vi "PixelFly.vi"() -> ()   [LabVIEW 2012]
uses:
  <vilib>/Platform/TimedLoop/XDataNode/timing_clust.ctl
  <vilib>/Platform/TimedLoop/XDataNode/nitl_modes.ctl
  <vilib>/Platform/TimedLoop/XDataNode/wakeup.ctl
  <vilib>/platform/TimedLoop/XDataNode/XDataNode.xnode
  <vilib>/Platform/TimedLoop/XDataNode/XDNodeRunTimeDep.lvlib
panel:
  in  "Tab Control":enum32{"Control", "Advanced"}(tab)
  out "Intensity Graph":u16[][](graph)
  in  "?":u16(ring) items=["Debug", "Bulb Trigger", "Free Run"]
  in  "bUseBuffer0":bool
  in  "Open StructureIn":T1={"Size"=88, "InterfaceType"=0, "Camera Number"=0, "CameraNumAtInterface"=0, "OpenFlags"=[], "OpenDWFlags"=[], "OpenPtrs"=[]}
  in  "bUseBuffer1":bool
  in  "stop":bool
  in  "stop 2":bool
  out "BufNr0":i16
  out "BufNr1":i16
  out "Bits/pixel":u16
  in  "ROIX1":u16=1 min=1
  in  "ROIY1":u16=1 min=1
  in  "ROIY0":u16=1 min=1
  in  "ROIX0":u16=1 min=1
  in  "DelayTimeBase":u16(ring)=2 items=["nanoseconds", "microseconds", "milliseconds"]
  in  "ExposureTimeBase":u16(ring)=1 items=["nanoseconds", "microseconds", "milliseconds"]
  in  "Exposure":u32=60
  in  "InterfaceType":u16(ring)=6 items=["IEEE1394 - Firewire", "IEEE1394/Firewire", "Matrox Helios Camera Link", "Silicon Software ME3 Camera Link", "National Instruments Camera Link", "Gigabit Ethernet", "USB", "Reserved", "Reserved", "Reserved", "Generic Camera Link with CLSER.DLL"]
  in  "Rate":i32
  in  "StorageMode":bool
  in  "TriggerMode":u16(ring)=2 items=["Auto", "Software", "External sequence start ", "External exposure control"]
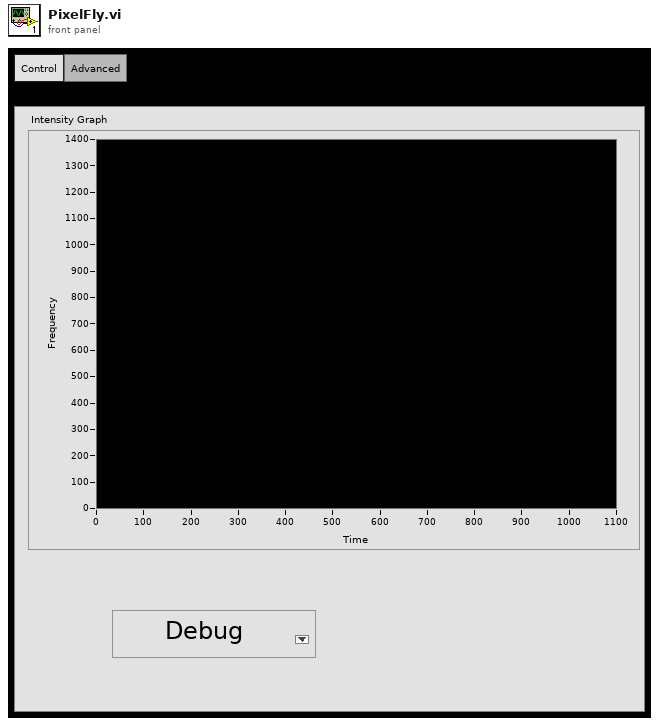
[diagram p1: front panel]
types:
  T1 = cluster{"Size":u16, "InterfaceType":u16, "Camera Number":u16, "CameraNumAtInterface":u16, "OpenFlags":u16[], "OpenDWFlags":u32[], "OpenPtrs":u32[]}
  T2 = typedef "XDNodeRunTimeDep.lvlib/timing_clust.ctl" = cluster{"Expected End [f-1]":u64, "Actual End [f-1]":u64, "Finished Late? [f-1]":bool, "Expected End [i-1]":u64, "Actual End [i-1]":u64, "Finished Late? [i-1]":bool, "Expected Start [i]":u64, "Actual Start [i]":u64, "Expected Start [f]":u64, "Actual Start [f]":u64, "Source Name":string, "Structure Name":string, "Period":i64, "Deadline":i64, "Offset":i64, "Start":i64, "Priority":i32, "Timeout":i32, "Mode":T3, "Wakeup Reason":T4, "Error":errorcluster, "Source Type":string, "Secondary Source Type":string, "Global End Time":u64, "Global Start Time":u64, "Frame Duration":u64, "Iteration Duration":u64, "Assigned CPU":i32, "I/O Scan Engine Mode":u32}
  T3 = typedef "XDNodeRunTimeDep.lvlib/nitl_modes.ctl" = enum32{"No Change", "Process missed periods, maintain original phase", "Discard missed periods, maintain original phase", "Process missed periods, ignore original phase", "Discard missed periods, ignore original phase"}
  T4 = typedef "XDNodeRunTimeDep.lvlib/wakeup.ctl" = enum32{"Normal", "Aborted", "Asynchronous wakeup", "Timing source error", "Timed loop error", "Timeout"}
  T5 = cluster{"Size":u16, "CamType":u16, "CamSubType":u16, "SerialNumber":u32, "HWVersion":u32, "FWVersion":u32, "InterfaceType":u16, "HardwareVersion":cluster{"BoardNum":u16, "HWVersions":cluster{"BoardName":string, "BatchNumber":u16, "MinorRevision":u8, "MajorRevision":u8, "Variant":u16}[]}, "FirmwareVersion":cluster{"DeviceNum":u16, "FWVersions":cluster{"DeviceName":string, "MinorRevision":u8, "MajorRevision":u8, "Variant":u16}[]}}
  T6 = cluster{"Size":u16, "SensorTypeDESC":u16, "SensorSubtypeDESC":u16, "MaxHorizontalResStdDESC":u16, "MaxVerticalResStdDESC":u16, "MaxHorizontalResExtDESC":u16, "MaxVerticalResExtDESC":u16, "DynResDESC":u16, "MaxBinHorzDESC":u16, "BinHorzStepDESC":bool, "MaxBinVertDESC":u16, "BinVertStepDESC":bool, "ROIHorzStepDESC":u16, "ROIVertStepDESC":u16, "NumADCDESC":u16, "IRDESC":bool, "MinDelayDESC":u32, "MaxDelayDESC":u32, "MinDelayStepDESC":u32, "MinExpoDESC":u32, "MaxExpoDESC":u32, "MinExpoStepDESC":u32, "MinDelayIRDESC":u32, "MaxDelayIRDESC":u32, "MinExpoIRDESC":u32, "MaxExpoIRDESC":u32, "TimeTableDESC":bool, "DoubleImageDESC":bool, "MinCoolSetDESC":i16, "MaxCoolSetDESC":i16, "MDefaultCoolSetDESC":i16, "PowerDownModeDESC":bool, "OffsetRegDESC":bool, "ColorPattern":cluster{"UpperLeftColor":u8, "UpperRightColor":u8, "LowerLeftColor":u8, "LowerRightColor":u8}, "PatternTypeDESC":bool, "PixelRates":u32[], "CoversionFactors":u16[], "Reserved":u32[], "NoiseFilterCapable":bool, "HotPixelCapable":bool, "HotPixelWithNoiseFilter":bool, "ASCIITimeCapable":bool, "Extended Description":bool, "Get Extended":bool, "Reserved Flag 1":bool, "Reserved Flag 2":bool}
  T7 = cluster{u16[][], "XResAct":u16, "YResAct":u16, "BufNrOut":i16, "BufNrOut":i16, "ErrorOut":errorcluster, "hout":u64, "Bits/pixel":u16}
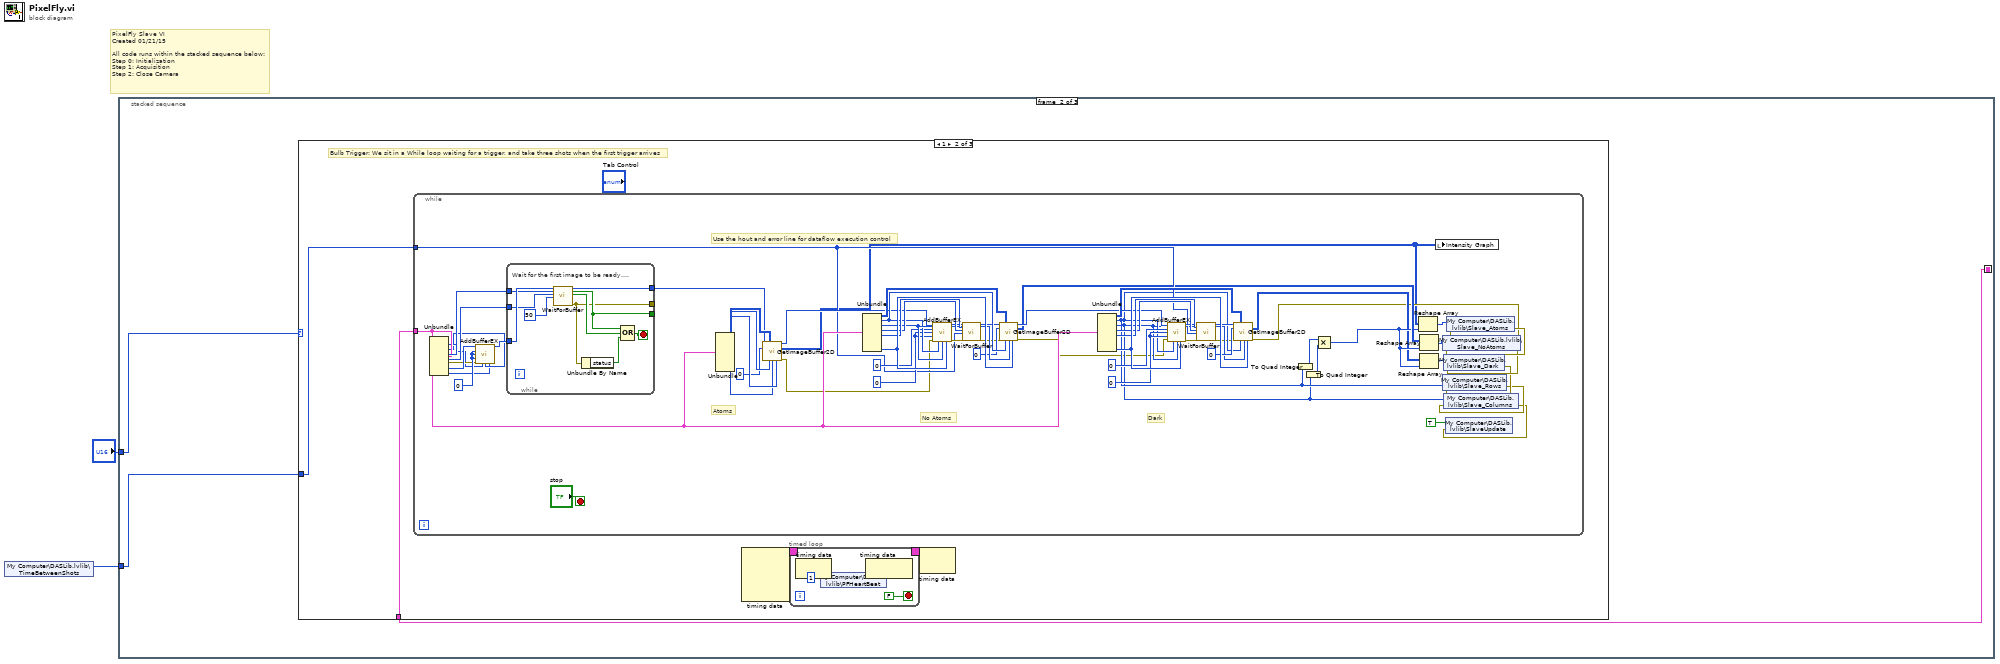
[diagram p0: block diagram]
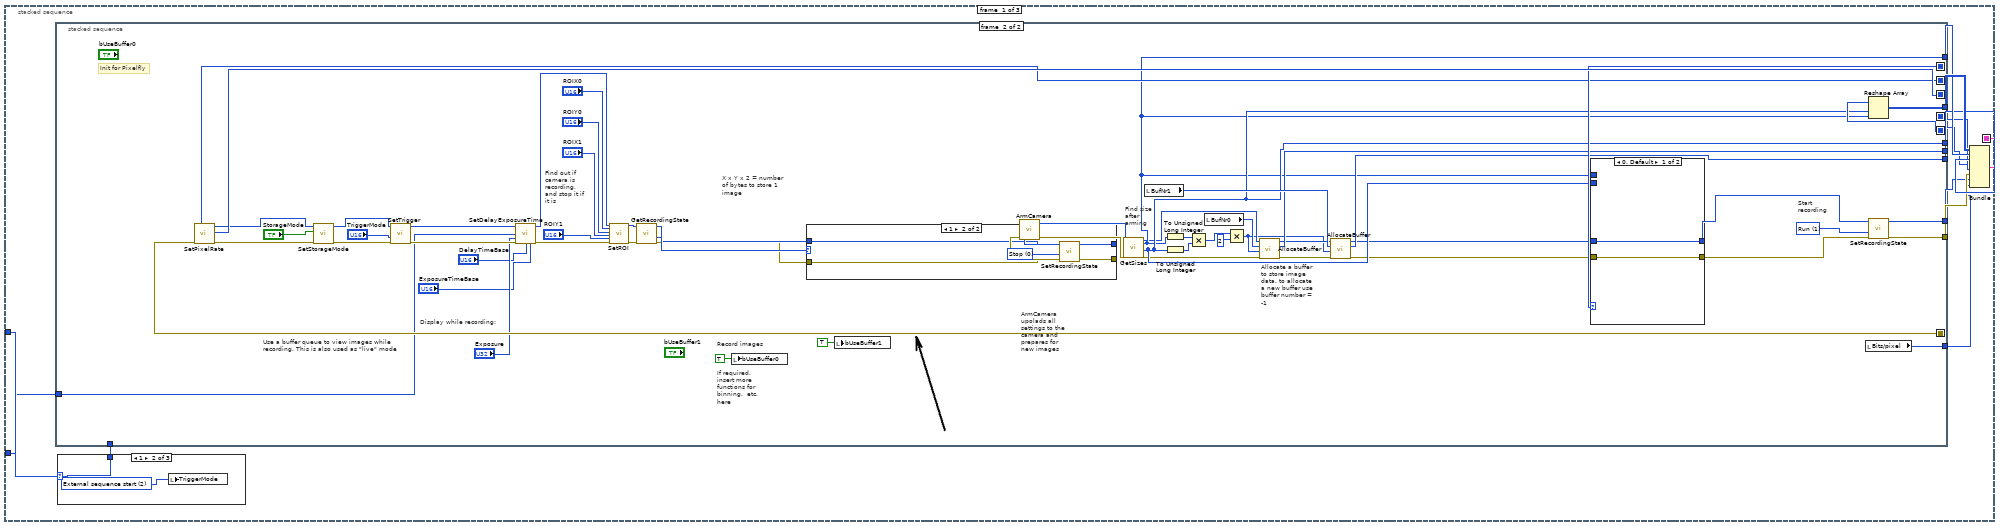
[diagram p2: hidden frame]
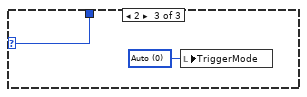
[diagram p4: hidden frame]
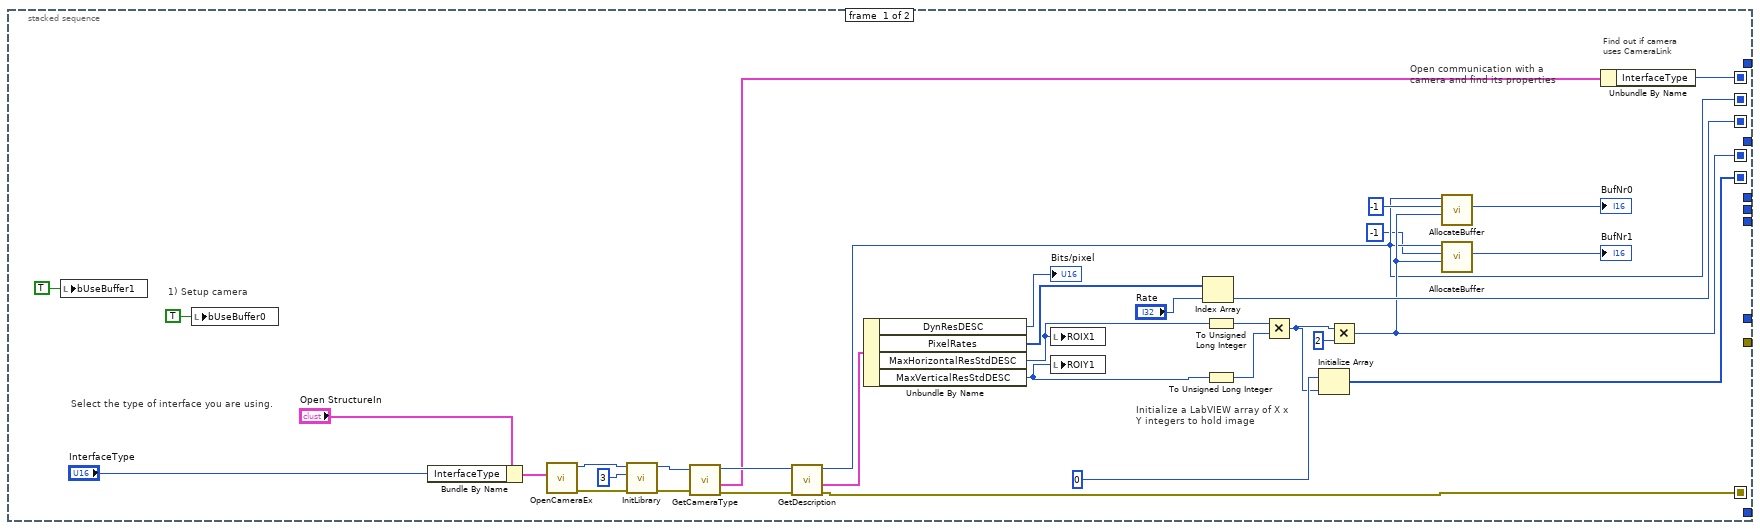
[diagram p5: hidden frame]
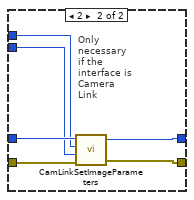
[diagram p6: hidden frame]
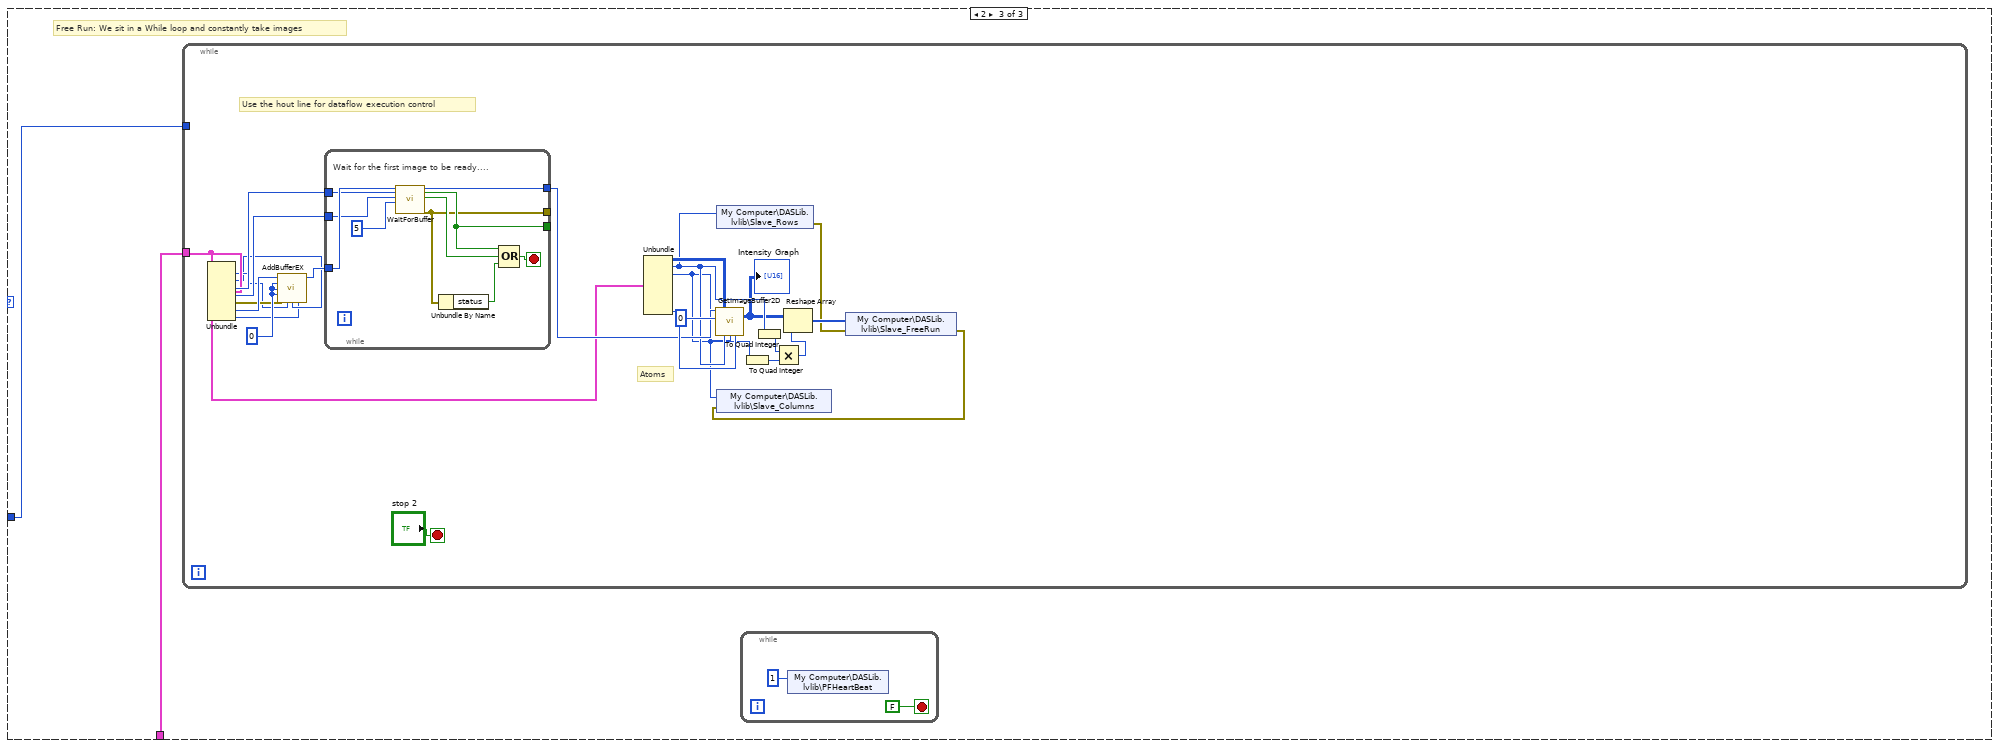
[diagram p9: hidden frame]
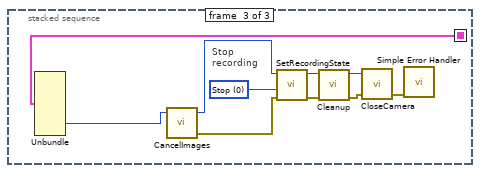
[diagram p10: hidden frame]
diagram:
  # "PixelFly Slave VI\nCreated 01/21/15\n\nAll code runs within the stacked sequence below:\nStep 0: Initialization\nStep 1: Acquisition\nStep 2: Close Camera"
  n1 = shared-variable "My Computer\\DASLib.lvlib\\TimeBetweenShots"() -> (w1:i64)  [unwired: 1 in, 1 out]
  n2 = stacked-sequence {
    seq-local: [w6 _ _] -> [_ w128 w253]
    tunnel: "?" -> [w5 w129 _]
    tunnel: w1 -> [w3 w127 _]
    frame #0 {
      n3 = case shown="1" w5 {
        selector: w5 -> [w15 w16 w18]
        tunnel: [w15 w16 w18] -> w4
        frame 0, Default {
        }
        frame 1 {
          w17 = u16 2 items=["Auto", "Software", "External sequence start ", "External exposure control"] ("TriggerMode")
          n4 = local write "TriggerMode"(w17) -> ()
        }
        frame 2 {
          w19 = u16 0 items=["Auto", "Software", "External sequence start ", "External exposure control"] ("TriggerMode")
          n5 = local write "TriggerMode"(w19) -> ()
        }
      }
      n6 = stacked-sequence {
        seq-local: [w50 _] -> [_ w108]
        seq-local: [w31 _] -> [_ _]
        seq-local: [w43 _] -> [_ w110]
        seq-local: [w30 _] -> [_ w105]
        seq-local: [w42 _] -> [_ w111]
        seq-local: [w41 _] -> [_ w109]
        tunnel: [_ w104] -> w14
        tunnel: [_ w100] -> w13
        tunnel: [_ w103] -> w12
        tunnel: [_ w102] -> w11
        tunnel: [_ w101] -> w10
        tunnel: [_ w99] -> w8
        tunnel: [_ w98] -> w9
        tunnel: [_ w97] -> w7
        tunnel: w4 -> [_ _]
        tunnel: w3 -> [_ w54]
        frame #0 {
          # "Select the type of interface you are using."
          # "1) Setup camera"
          # "Find out if camera uses CameraLink"
          # "Initialize a LabVIEW array of X x Y integers to hold image"
          # "Open communication with a camera and find its properties"
          n7 = local write "bUseBuffer1"(TRUE) -> ()
          n8 = local write "bUseBuffer0"(TRUE) -> ()
          n9 = Bundle By Name(cluster="Open StructureIn", "InterfaceType"="InterfaceType") -> (w38:T1)
          n10 = call "OpenCameraEx.vi"("OpenStructureIn"=w38) -> ("error out"=w22:errorcluster, "hout"=w23:u64)  [unwired: 3 in, 2 out]
          n11 = call "InitLibrary.vi"("error in (no error)"=w22, "InterfaceType"=u32 3, "ph"=w23) -> ("error out"=w20:errorcluster, "hout"=w21:u64)  [unwired: 7 in]
          n12 = call "GetCameraType.vi"("ph"=w21, "error in (no error)"=w20) -> ("hout"=w47:u64, "CameraType"=w45:T5, "error out"=w46:errorcluster)  [unwired: 1 in, 1 out]
          n13 = call "GetDescription.vi"("ErrorIn"=w46, "ph"=w47) -> ("ErrorOut"=w42:errorcluster, "Description"=w49:T6, "hout"=w30:u64)  [unwired: 2 in, 1 out]
          n14 = Unbundle By Name(w49) -> ("DynResDESC"=→"Bits/pixel":u16, "PixelRates"=w44:u32[], "MaxHorizontalResStdDESC"=w36:u16, "MaxVerticalResStdDESC"=w35:u16)
          n15 = local write "ROIX1"(w36) -> ()
          n16 = local write "ROIY1"(w35) -> ()
          n17 = Index Array(array=w44, index="Rate") -> (element=w43:u32)
          n18 = To Unsigned Long Integer(number=w36) -> (unsigned 32bit integer=w33:u32)
          n19 = To Unsigned Long Integer(number=w35) -> (unsigned 32bit integer=w32:u32)
          n20 = Multiply(x=w33, y=w32) -> (x*y=w51:u32)
          n21 = Initialize Array(u16 0 ("Element Data"), w51) -> (w50:u16[])
          n22 = Multiply(x=w51, y=u32 2) -> (x*y=w31:u32)
          n23 = call "AllocateBuffer.vi"("Size"=w31, "BufNr"=i16 -1, "ph"=w30) -> ("BufNrOut"=→"BufNr0":i16)  [unwired: 3 in, 5 out]
          n24 = call "AllocateBuffer.vi"("Size"=w31, "BufNr"=-1, "ph"=w30) -> ("BufNrOut"=→"BufNr1":i16)  [unwired: 3 in, 5 out]
          n25 = Unbundle By Name(w45) -> ("InterfaceType"=w41:u16)
        }
        frame #1 {
          w96 = u16 1 items=["Stop", "Run"] ("RecordingState")
          # "Init for Pixelfly"
          # "Record images"
          # "Start recording"
          # "Allocate a buffer to store image data. to allocate a new buffer use buffer number = -1"
          # "Find size after arming"
          # "ArmCamera upolads all settings to the camera and prepares for new images"
          # "Find out if camera is recording, and stop it if it is"
          # "If required, insert more functions for binning.  etc. here"
          # "X x Y x 2 = number of bytes to store 1 image"
          # "Use a buffer queue to view images while recording. This is also used as \"live\" mode"
          # "Display while recording:"
          n26 = call "SetPixelRate.vi"("error in (no error)"=w111, "PixelRate"=w110, "ph"=w105) -> ("error out"=w94:errorcluster, "hout"=w95:u64)  [unwired: 2 in, 1 out]
          n27 = call "SetStorageMode.vi"("error in (no error)"=w94, "StorageMode"="StorageMode", "ph"=w95) -> ("error out"=w86:errorcluster, "hout"=w87:u64)  [unwired: 2 in, 1 out]
          n28 = call "SetTrigger.vi"("error in (no error)"=w86, "TriggerMode"="TriggerMode", "ph"=w87) -> ("error out"=w79:errorcluster, "hout"=w80:u64)  [unwired: 2 in, 1 out]
          n29 = call "SetDelayExposureTime.vi"("ph"=w80, "Delay"=w54, "Exposure"="Exposure", "error in (no error)"=w79, "DelayTimeBase"="DelayTimeBase", "ExposureTimeBase"="ExposureTimeBase") -> ("hout"=w69:u64, "error out"=w67:errorcluster)  [unwired: 7 in, 1 out]
          n30 = call "SetROI.vi"("ph"=w69, "ROIX0"="ROIX0", "ROIY0"="ROIY0", "ROIX1"="ROIX1", "ROIY1"="ROIY1", "error in (no error)"=w67) -> ("hout"=w68:u64, "error out"=w66:errorcluster)  [unwired: 12 in]
          n31 = call "GetRecordingState.vi"("ErrorIn"=w66, "ph"=w68) -> ("ErrorOut"=w90:errorcluster, "RecordingState"=w92:u16, "hout"=w91:u64)  [unwired: 2 in, 1 out]
          n32 = local write "bUseBuffer0"(TRUE) -> ()
          n33 = case shown="1" w92 {
            tunnel: w91 -> [w121 w125]
            tunnel: w90 -> [w120 w124]
            tunnel: [w121 w123] -> w89
            tunnel: [w120 w122] -> w88
            frame 0, Default {
            }
            frame 1 {
              w126 = u16 0 items=["Stop", "Run"] ("RecordingState")
              n34 = call "SetRecordingState.vi"("ErrorIn"=w124, "RecordingState"=w126, "ph"=w125) -> ("ErrorOut"=w122:errorcluster, "hout"=w123:u64)  [unwired: 2 in, 1 out]
            }
          }
          n35 = local write "bUseBuffer1"(TRUE) -> ()
          n36 = call "ArmCamera.vi"("error in (no error)"=w88, "ph"=w89) -> ("error out"=w84:errorcluster, "hout"=w85:u64)  [unwired: 1 in, 1 out]
          n37 = call "GetSizes.vi"("ph"=w85, "ErrorIn"=w84) -> ("hout"=w81:u64, "XResAct"=w100:u16, "YResAct"=w103:u16, "ErrorOut"=w83:errorcluster)  [unwired: 11 in, 3 out]
          n38 = local read "BufNr1"() -> (w107:i16)
          n39 = To Unsigned Long Integer(number=w100) -> (unsigned 32bit integer=w70:u32)
          n40 = To Unsigned Long Integer(number=w103) -> (unsigned 32bit integer=w71:u32)
          n41 = Multiply(x=w70, y=w71) -> (x*y=w72:u32)
          n42 = local read "BufNr0"() -> (w106:i16)
          n43 = Multiply(x=w72, y=u32 2) -> (x*y=w57:u32)
          n44 = call "AllocateBuffer.vi"("error in (no error)"=w83, "Size"=w57, "BufNr"=w106, "ph"=w81) -> ("error out"=w61:errorcluster, "BufNrOut"=w102:i16, "hout"=w59:u64)  [unwired: 2 in, 3 out]
          n45 = call "AllocateBuffer.vi"("error in (no error)"=w61, "Size"=w57, "BufNr"=w107, "ph"=w59) -> ("error out"=w60:errorcluster, "BufNrOut"=w101:i16, "hout"=w58:u64)  [unwired: 2 in, 3 out]
          n46 = case shown="0, Default" w109 {
            tunnel: w60 -> [w112 w119]
            tunnel: [w112 w118] -> w75
            tunnel: w58 -> [w113 w117]
            tunnel: [w113 w116] -> w74
            tunnel: w103 -> [_ w115]
            tunnel: w100 -> [_ w114]
            frame 0, Default {
            }
            frame 2 {
              # "Only necessary if the interface is Camera Link"
              n47 = call "CamLinkSetImageParameters.vi"("error in (no error)"=w119, "YRes"=w115, "XRes"=w114, "ph"=w117) -> ("error out"=w118:errorcluster, "hout"=w116:u64)  [unwired: 1 out]
            }
          }
          n48 = local read "Bits/pixel"() -> (w97:u16)
          n49 = Reshape Array(w108, w103, w100) -> (w104:u16[][])
          n50 = call "SetRecordingState.vi"("ErrorIn"=w75, "RecordingState"=w96, "ph"=w74) -> ("ErrorOut"=w98:errorcluster, "hout"=w99:u64)  [unwired: 2 in, 1 out]
        }
      }
      n51 = Bundle(w14, "XResAct"=w13, "YResAct"=w12, "BufNrOut"=w10, "BufNrOut"=w11, "ErrorOut"=w9, "hout"=w8, "Bits/pixel"=w7) -> (w6:T7)  [unwired: 1 in]
    }
    frame #1 {
      n52 = case shown="1" w129 {
        tunnel: w128 -> [_ w133 w215]
        tunnel: w127 -> [_ w132 w214]
        frame 0, Default {
          # "Debug Mode: Do nothing here\nProceeds directly to closing the camera"
        }
        frame 1 {
          # "Bulb Trigger: We sit in a While loop waiting for a trigger, and take three shots when the first trigger arrives"
          n53 = while {
            tunnel: w133 -> [w166]
            tunnel: w132 -> [w165]
            stop <- "stop" stop-if-true
            w171 = 0
            w182 = 0
            w198 = 0
            # "Dark"
            # "No Atoms"
            # "Atoms"
            # "Use the hout and error line for dataflow execution control"
            n54 = Unbundle(w166) -> ("XResAct"=w164:u16, "YResAct"=w163:u16, "BufNrOut"=w194:i16, "BufNrOut"=w193:i16, "ErrorOut"=w196:errorcluster, "hout"=w197:u64, "Bits/pixel"=w162:u16)  [unwired: 1 out]
            n55 = call "AddBufferEX.vi"("ph"=w197, "BuffNr"=w198, "1stImage"=w198, "LastImage"=w198, "error in (no error)"=w196, "XRes"=w164, "YRes"=w163, "BitPerPixel"=w162) -> ("hout"=w195:u64)  [unwired: 5 in, 2 out]
            n56 = while {
              tunnel: [w209] -> _
              tunnel: [w212] -> _
              tunnel: w195 -> [w207]
              tunnel: w194 -> [w206]
              tunnel: w193 -> [w205]
              tunnel: [w204] -> w192
              stop <- w213 stop-if-true
              # "Wait for the first image to be ready...."
              n57 = call "WaitForBuffer.vi"("ph"=w207, "sBufNr"=w206, "sBufNr 2"=w205, "timeout"=50) -> ("hout"=w204:u64, "Buffer_Ready"=w212:bool, "Buffer_Ready 2"=w211:bool, "error out"=w209:errorcluster)  [unwired: 11 in, 1 out]
              n58 = Unbundle By Name(w209) -> ("status"=w208:bool)
              n59 = Compound Arithmetic op=OR(w212, w211, w208) -> (w213:bool)
            }
            n60 = Unbundle(w166) -> (w203:u16[][], "XResAct"=w201:u16, "YResAct"=w191:u16, "Bits/pixel"=w202:u16)  [unwired: 4 out]
            n61 = call "GetImageBuffer2D.vi"("ph"=w192, "BuffIn"=w203, "BuffNr"=i16 0, "xRes"=w201, "yRes"=w191, "Bitresolution"=w202) -> ("hout"=w178:u64, "BuffOut"=w140:u16[][], "error out"=w152:errorcluster)  [unwired: 6 in, 1 out]
            n62 = Unbundle(w166) -> (w190:u16[][], "XResAct"=w185:u16, "YResAct"=w186:u16, "BufNrOut"=w187:i16, "BufNrOut"=w188:i16, "Bits/pixel"=w189:u16)  [unwired: 2 out]
            n63 = call "AddBufferEX.vi"("ph"=w178, "BuffNr"=i16 0, "1stImage"=w182, "LastImage"=w182, "error in (no error)"=w152, "XRes"=w185, "YRes"=w186, "BitPerPixel"=w189) -> ("hout"=w180:u64, "error out"=w181:errorcluster)  [unwired: 5 in, 1 out]
            n64 = call "WaitForBuffer.vi"("ph"=w180, "sBufNr"=w188, "sBufNr 2"=w187, "timeout"=w165, "error in (no error)"=w181) -> ("hout"=w179:u64, "error out"=w153:errorcluster)  [unwired: 10 in, 3 out]
            n65 = call "GetImageBuffer2D.vi"("ph"=w179, "BuffIn"=w190, "BuffNr"=i16 0, "error in (no error)"=w153, "xRes"=w185, "yRes"=w186, "Bitresolution"=w189) -> ("hout"=w167:u64, "BuffOut"=w161:u16[][], "error out"=w151:errorcluster)  [unwired: 5 in, 1 out]
            n66 = Unbundle(w166) -> (w177:u16[][], "XResAct"=w160:u16, "YResAct"=w159:u16, "BufNrOut"=w174:i16, "BufNrOut"=w175:i16, "Bits/pixel"=w176:u16)  [unwired: 2 out]
            n67 = call "AddBufferEX.vi"("ph"=w167, "BuffNr"=i16 0, "1stImage"=w171, "LastImage"=w171, "error in (no error)"=w151, "XRes"=w160, "YRes"=w159, "BitPerPixel"=w176) -> ("hout"=w169:u64, "error out"=w170:errorcluster)  [unwired: 5 in, 1 out]
            n68 = call "WaitForBuffer.vi"("ph"=w169, "sBufNr"=w175, "sBufNr 2"=w174, "timeout"=w165, "error in (no error)"=w170) -> ("hout"=w168:u64, "error out"=w150:errorcluster)  [unwired: 10 in, 3 out]
            n69 = call "GetImageBuffer2D.vi"("ph"=w168, "BuffIn"=w177, "BuffNr"=i16 0, "error in (no error)"=w150, "xRes"=w160, "yRes"=w159, "Bitresolution"=w176) -> ("BuffOut"=w154:u16[][], "error out"=w148:errorcluster)  [unwired: 5 in, 2 out]
            n70 = To Quad Integer(1:w160) -> (0:w141:i64)
            n71 = To Quad Integer(1:w159) -> (0:w142:i64)
            n72 = Multiply(x=w141, y=w142) -> (x*y=w158:i64)
            n73 = Reshape Array(w140, w158) -> (w157:u16[])
            n74 = Reshape Array(w161, w158) -> (w156:u16[])
            n75 = Reshape Array(w154, w158) -> (w155:u16[])
            n76 = local write "Intensity Graph"(w140) -> ()
            n77 = shared-variable "My Computer\\DASLib.lvlib\\Slave_Atoms"(w157, error in=w148) -> (error out=w149:errorcluster)
            n78 = shared-variable "My Computer\\DASLib.lvlib\\Slave_NoAtoms"(w156, error in=w149) -> (error out=w147:errorcluster)
            n79 = shared-variable "My Computer\\DASLib.lvlib\\Slave_Dark"(w155, error in=w147) -> (error out=w146:errorcluster)
            n80 = shared-variable "My Computer\\DASLib.lvlib\\Slave_Rows"(w160, error in=w146) -> (error out=w145:errorcluster)
            n81 = shared-variable "My Computer\\DASLib.lvlib\\Slave_Columns"(w159, error in=w145) -> (error out=w143:errorcluster)
            n82 = shared-variable "My Computer\\DASLib.lvlib\\SlaveUpdate"(TRUE ("SlaveUpdate"), error in=w143) -> ()  [unwired: 1 out]
          }
          n83 = node-c288() -> (w131:T2)  [unwired: 4 in]
          n84 = timed-loop {
            timing: w131 -> [_]
            timing-out: [_] -> w130
            stop <- FALSE stop-if-true
            n85 = node-c288() -> ()  [unwired: 1 in, 1 out]
            n86 = shared-variable "My Computer\\DASLib.lvlib\\PFHeartBeat"(i16 1 ("PFHeartBeat")) -> ()  [unwired: 1 in, 1 out]
            n87 = node-c288() -> ()  [unwired: 1 in, 1 out]
          }
          n88 = node-c288(w130) -> ()  [unwired: 1 out]
        }
        frame 2 {
          # "Free Run: We sit in a While loop and constantly take images"
          n89 = while {
            tunnel: w215 -> [w230]
            tunnel: w214 -> [_]
            stop <- "stop 2" stop-if-true
            w237 = 0
            # "Atoms"
            # "Use the hout line for dataflow execution control"
            n90 = Unbundle(w230) -> ("XResAct"=w229:u16, "YResAct"=w228:u16, "BufNrOut"=w233:i16, "BufNrOut"=w232:i16, "ErrorOut"=w235:errorcluster, "hout"=w236:u64, "Bits/pixel"=w227:u16)  [unwired: 1 out]
            n91 = call "AddBufferEX.vi"("ph"=w236, "BuffNr"=w237, "1stImage"=w237, "LastImage"=w237, "error in (no error)"=w235, "XRes"=w229, "YRes"=w228, "BitPerPixel"=w227) -> ("hout"=w234:u64)  [unwired: 5 in, 2 out]
            n92 = while {
              tunnel: [w247] -> _
              tunnel: [w250] -> _
              tunnel: w234 -> [w245]
              tunnel: w233 -> [w244]
              tunnel: w232 -> [w243]
              tunnel: [w242] -> w231
              stop <- w251 stop-if-true
              # "Wait for the first image to be ready...."
              n93 = call "WaitForBuffer.vi"("ph"=w245, "sBufNr"=w244, "sBufNr 2"=w243, "timeout"=5) -> ("hout"=w242:u64, "Buffer_Ready"=w250:bool, "Buffer_Ready 2"=w249:bool, "error out"=w247:errorcluster)  [unwired: 11 in, 1 out]
              n94 = Unbundle By Name(w247) -> ("status"=w246:bool)
              n95 = Compound Arithmetic op=OR(w250, w249, w246) -> (w251:bool)
            }
            n96 = Unbundle(w230) -> (w241:u16[][], "XResAct"=w225:u16, "YResAct"=w224:u16, "Bits/pixel"=w240:u16)  [unwired: 4 out]
            n97 = call "GetImageBuffer2D.vi"("ph"=w231, "BuffIn"=w241, "BuffNr"=i16 0, "xRes"=w225, "yRes"=w224, "Bitresolution"=w240) -> ("BuffOut"=w222:u16[][])  [unwired: 6 in, 3 out]
            "Intensity Graph" <- w222
            n98 = shared-variable "My Computer\\DASLib.lvlib\\Slave_Rows"(w225) -> (error out=w221:errorcluster)  [unwired: 1 in]
            n99 = To Quad Integer(1:w224) -> (0:w218:i64)
            n100 = To Quad Integer(1:w225) -> (0:w219:i64)
            n101 = Multiply(x=w219, y=w218) -> (x*y=w226:i64)
            n102 = Reshape Array(w222, w226) -> (w223:u16[])
            n103 = shared-variable "My Computer\\DASLib.lvlib\\Slave_FreeRun"(w223, error in=w221) -> (error out=w220:errorcluster)
            n104 = shared-variable "My Computer\\DASLib.lvlib\\Slave_Columns"(w224, error in=w220) -> ()  [unwired: 1 out]
          }
          n105 = while {
            stop <- FALSE stop-if-true
            n106 = shared-variable "My Computer\\DASLib.lvlib\\PFHeartBeat"(i16 1 ("PFHeartBeat")) -> ()  [unwired: 1 in, 1 out]
          }
        }
      }
    }
    frame #2 {
      w259 = u16 0 items=["Stop", "Run"] ("RecordingState")
      # "Stop recording"
      n107 = Unbundle(w253) -> ("hout"=w252:u64)  [unwired: 7 out]
      n108 = call "CancelImages.vi"("ph"=w252) -> ("error out"=w261:errorcluster, "hout"=w260:u64)  [unwired: 2 in, 1 out]
      n109 = call "SetRecordingState.vi"("ErrorIn"=w261, "RecordingState"=w259, "ph"=w260) -> ("ErrorOut"=w254:errorcluster, "hout"=w255:u64)  [unwired: 2 in, 1 out]
      n110 = call "Cleanup.vi"("error in (no error)"=w254, "ph"=w255) -> ("error out"=w257:errorcluster, "hout"=w256:u64)  [unwired: 8 in]
      n111 = call "CloseCamera.vi"("ErrorIn"=w257, "Handle in"=w256) -> ("ErrorOut"=w258:errorcluster)  [unwired: 1 in, 2 out]
      n112 = call <vilib>:"Simple Error Handler.vi"("error in (no error)"=w258) -> ()  [unwired: 4 in, 5 out]
    }
  }
